vi "Write Trig Src Ref.vi"(8 "error in":errorcluster, 10 "Trig Src Ref":refnum<vi>, 11 "AnalogInput in":refnum<class "AnalogInput.lvclass">) -> (0 "error out":errorcluster, 3 "AnalogInput out":refnum<class "AnalogInput.lvclass">)   [LabVIEW 2019, in "AnalogInput.lvlib" / "AnalogInput.lvclass"]
uses:
  Library/AnalogInput.lvclass
  Library/AnalogInput.lvclass/AnalogInput.ctl
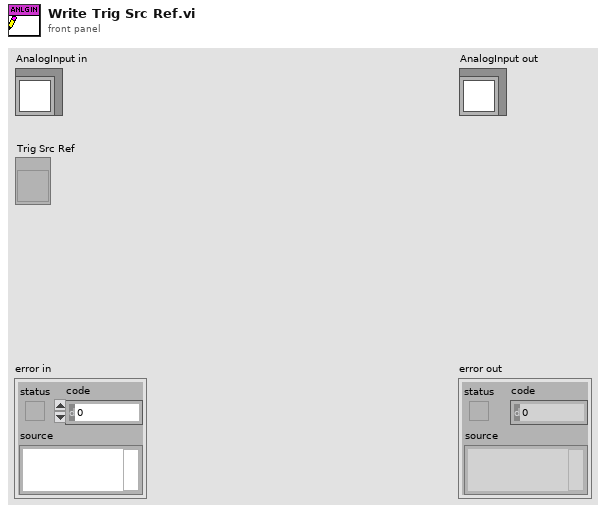
[diagram p1: front panel]
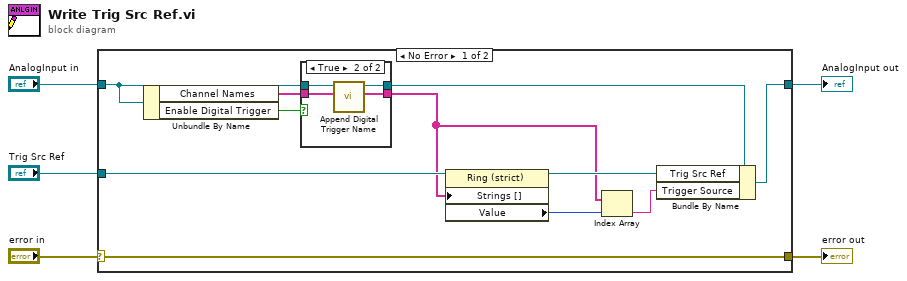
[diagram p0: block diagram]
diagram:
  n1 = case shown="No Error" "error in" {
    selector: "error in" -> [w16 w23]
    tunnel: [w16 w23] -> w4
    tunnel: [w15 w24] -> w2
    tunnel: "AnalogInput in" -> [w10 w24]
    tunnel: "Trig Src Ref" -> [w14 _]
    frame No Error {
      n2 = Unbundle By Name(w10) -> ("Channel Names"=w8:string[], "Enable Digital Trigger"=w6:bool)
      n3 = case shown="True" w6 {
        tunnel: w10 -> [w18 w22]
        tunnel: [w18 w21] -> w9
        tunnel: w8 -> [w17 w20]
        tunnel: [w17 w19] -> w7
        frame False {
        }
        frame True {
          n4 = call "Append Digital Trigger Name.vi"("Channels In"=w20, "AnalogInput in"=w22) -> ("Channels Out"=w19:string[], "AnalogInput out"=w21:refnum<class "AnalogInput.lvclass">)  [unwired: 7 in, 1 out]
        }
      }
      n5 = property class="Ring (strict)"(reference=w14, "Strings []"=w7) -> (reference out=w13:refnum<vi>, "Value"=w12:u16)  [unwired: 1 in, 1 out]
      n6 = Index Array(array=w7, index=w12) -> (element=w11:string)
      n7 = Bundle By Name(cluster=w9, "Trig Src Ref"=w13, "Trigger Source"=w11) -> (w15:refnum<class "AnalogInput.lvclass">)
    }
    frame Error {
    }
  }
  "error out" <- w4
  "AnalogInput out" <- w2
